vi "Interface_Asset_Update Tags.vi"(8 "error in (no error)":errorcluster, 10 "TagBus DVR":refnum<data-value>, 11 "Asset_Interface in":refnum<class "EnergyStorage.lvclass">) -> (0 "error out":errorcluster, 2 "TagBus DVR out":refnum<data-value>, 3 "Asset_Interface out":refnum<class "EnergyStorage.lvclass">)   [LabVIEW 2015, in "EnergyStorage.lvclass"]
uses:
  EnergyStorage.lvclass
  EnergyStorage_Status.ctl
  TagBus/TagBus.lvclass
  EnergyStorage.lvclass/EnergyStorage.ctl
panel:
  out "Status":T1
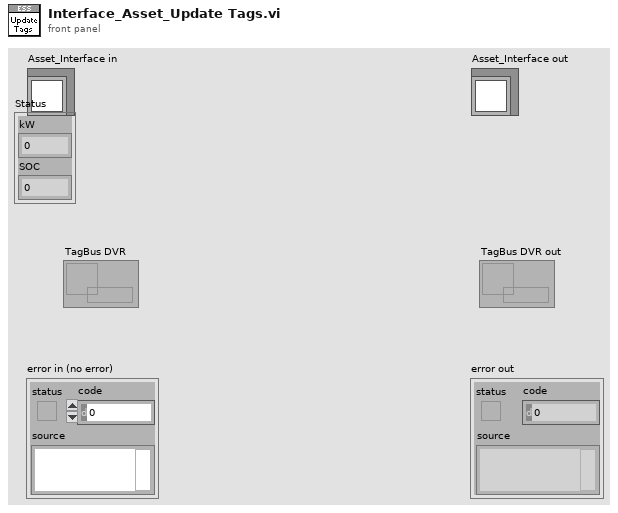
[diagram p1: front panel]
types:
  T1 = typedef "EnergyStorage.lvclass/EnergyStorage_Status.ctl" = cluster{"kW":dbl, "SOC":dbl}
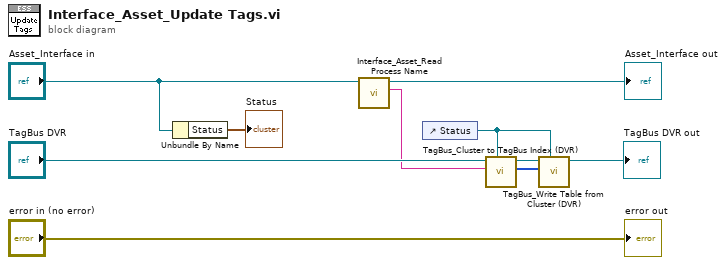
[diagram p0: block diagram]
diagram:
  n1 = Unbundle By Name("Asset_Interface in") -> ("Status"=→"Status":T1)
  n2 = call-dynamic "Interface_Asset_Read Process Name.vi"("EnergyStorage in"="Asset_Interface in") -> ("Process Name"=w2:string, "EnergyStorage out"=→"Asset_Interface out":refnum<class "EnergyStorage.lvclass">)  [unwired: 9 in]
  n3 = control-ref of="Status"() -> (w4:refnum<vi>)
  n4 = call "TagBus_Cluster to TagBus Index (DVR).vi"("Clust Refnum"=w4, "Tag Name Prepend"=w2, "TagBus DVR"="TagBus DVR") -> ("Index Array"=w5:i32[], "TagBus DVR out"=w6:refnum<data-value>)  [unwired: 7 in]
  n5 = call "TagBus_Write Table from Cluster (DVR).vi"("Clust Refnum"=w4, "Index Array"=w5, "Data Value Reference in"=w6) -> ("Data Value Reference out"=→"TagBus DVR out":refnum<data-value>)  [unwired: 8 in]
  "error out" <- "error in (no error)"
